vi "HTVacuum.destructor.vi"(0 "i ref in":refnum<vi>, 5 "error in (no error)":errorcluster) -> (19 "error out":errorcluster)   [LabVIEW 2014, in "HTVacuum.lvlib"]
doc: "This is the destructor of a class.\n\nLicense Agreement for this software:\n\nCopyright (C)\nGesellschaft für Schwerionenforschung, GSI\nPlanckstr. 1\n64291 Darmstadt\nGermany\n\nContact: D.Beck@gsi.de \n\nThis program is free software; you can redistribute it and/or modify it under the terms of the \nGNU General Public License as published by the Free Software Foundation; either version 2 of \nthe license, or (at your option) any later version.\n\nThis program is distributed in the hope that it will be useful, but WITHOUT ANY WARRANTY; \nwithout even the implied warranty of MERCHANTABILITY or FITNESS FOR A PARTICULAR PURPOSE. See the GNU General License for more details (http://www.gnu.org).\n\nGesellschaft für Schwerionenforschung, GSI\nPlanckstr. 1, 64291 Darmstadt, Germany\nFor all questions and ideas contact: M.Richter@gsi.de, H.Brand@gsi.de or D.Beck@gsi.de.\nLast update: 16-JUN-2004"
uses:
  HTVacuum.lvlib
  instr.lib/M&M/M&M/_ica01/ica-Lib SubVIs/M&M SubVIs/M&M USB close.vi
  CS_Core/BaseProcess/BaseProcess.lvlib
  CS_Core/CSApplicationBaseClasses/DeviceBase/DeviceBase.lvlib
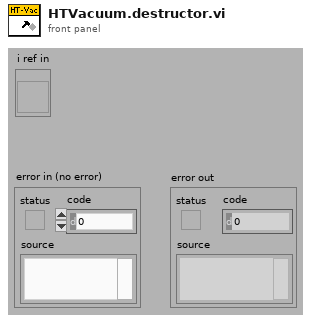
[diagram p1: front panel]
types:
  T1 = typedef "HTVacuum.lvlib/HTVacuum.i attribute.ctl" = cluster{"USB-Handle":cluster{"Write handle":i32, "Read handle":i32}}
  T2 = enum16{"SetAttribute", "GetAttribute", "CreateAttribute", "DestroyAttribute", "DestroyAllAtributes"}
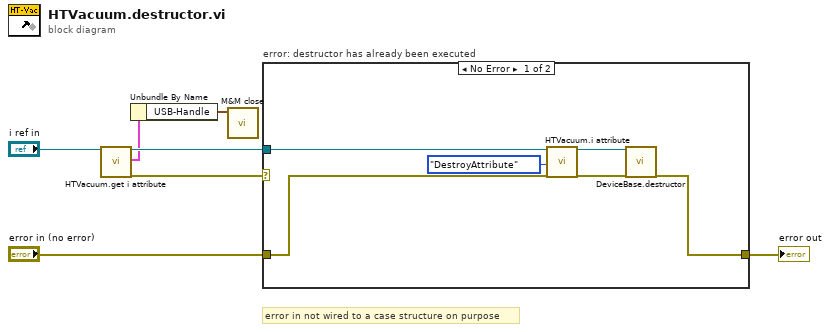
[diagram p0: block diagram]
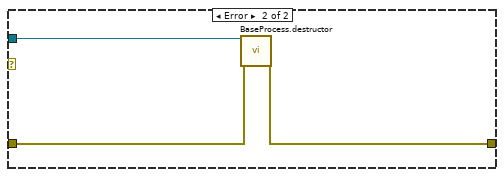
[diagram p2: hidden frame]
diagram:
  # "error in not wired to a case structure on purpose"
  n1 = call "HTVacuum.get i attribute.vi"("i ref in"="i ref in") -> ("i ref out"=w3:refnum<vi>, "i attribute"=w2:T1, "error out"=w4:errorcluster)  [unwired: 16 in]
  n2 = Unbundle By Name(w2) -> ("USB-Handle"=w1:cluster{"Write handle":i32, "Read handle":i32})
  n3 = call-poly "M&M close.vi"("Handles in"=w1) -> ()  [unwired: 9 in, 2 out]
  n4 = case "error: destructor has already been executed" shown="No Error" w4 {
    tunnel: [w8 w14] -> w7
    tunnel: "error in (no error)" -> [w12 w15]
    tunnel: w3 -> [w11 w16]
    frame No Error {
      n5 = call "HTVacuum.i attribute.vi"("VI Refnum"=w11, "Action"=T2."DestroyAttribute", "error in (no error)"=w12) -> ("VI Refnum out"=w10:refnum<vi>, "error out"=w9:errorcluster)  [unwired: 14 in, 1 out]
      n6 = call "DeviceBase.destructor.vi"("i ref in"=w10, "error in (no error)"=w9) -> ("error out"=w8:errorcluster)  [unwired: 17 in]
    }
    frame Error {
      n7 = call "BaseProcess.destructor.vi"("i ref in"=w16, "error in (no error)"=w15) -> ("error out"=w14:errorcluster)  [unwired: 17 in]
    }
  }
  "error out" <- w7
